vi "Read Monitor Resolution.vi"(8 "error in (no error)":errorcluster) -> (0 "error out":errorcluster, 2 "Monitor Resolution":cluster{"H":i16, "V":i16}[](array[cluster]), 3 "Number of Displays":i32)   [LabVIEW 2020, in "MacroAssert.lvlib"]
doc: "This will return an array of clusters with the Horizontal and verticle dimensions in pixels for each display."
uses:
  MacroAssert.lvlib
  System.Windows.Forms
  System.Drawing
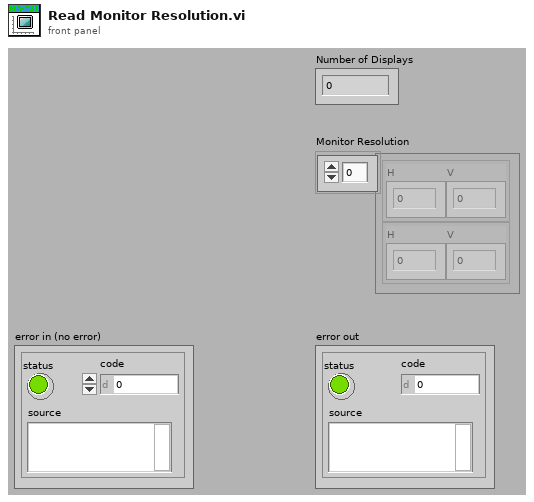
[diagram p1: front panel]
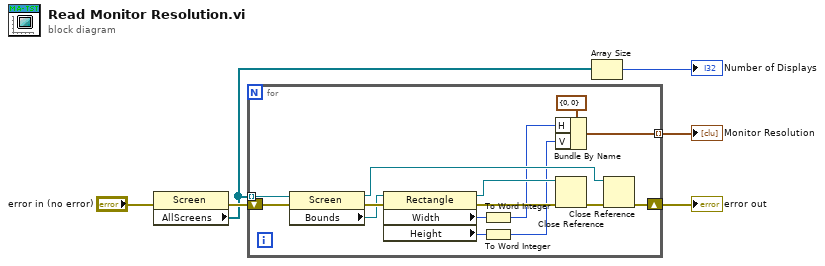
[diagram p0: block diagram]
diagram:
  n1 = property class="Screen"(error in="error in (no error)") -> (error out=w6:errorcluster, "AllScreens"=w4:refnum<k24>[])  [unwired: 1 in, 1 out]
  n2 = for {
    tunnel: w4 -> [w19] mode=indexing
    shift-right: [w11] -> w1
    shift-left: w6 -> [w21]
    tunnel: [w14] -> w2 mode=indexing
    n3 = property class="Screen"(reference=w19, error in=w21) -> (reference out=w9:refnum<k24>, error out=w20:errorcluster, "Bounds"=w18:refnum<k24>)
    n4 = property class="Rectangle"(reference=w18, error in=w20) -> (reference out=w10:refnum<k24>, error out=w13:errorcluster, "Width"=w15:i32, "Height"=w16:i32)
    n5 = To Word Integer(number=w15) -> (16bit integer=w8:i16)
    n6 = To Word Integer(number=w16) -> (16bit integer=w7:i16)
    n7 = Bundle By Name(cluster=cluster{"V":i16, "H":i16} {"V"=0, "H"=0} ("input cluster"), "H"=w8, "V"=w7) -> (w14:cluster{"V":i16, "H":i16})
    n8 = Close Reference(reference=w10, error in (no error)=w13) -> (error out=w12:errorcluster)
    n9 = Close Reference(reference=w9, error in (no error)=w12) -> (error out=w11:errorcluster)
  }
  "error out" <- w1
  "Monitor Resolution" <- w2
  n10 = Array Size(array=w4) -> (size(s)=→"Number of Displays":i32)
